vi "Get SysDef Path.vi"(11 "Scalar Channels Testing in":refnum<class "FPGA Addon Test Class.lvclass">) -> (2 "SysDef Path":path, 3 "Scalar Channels Testing out":refnum<class "FPGA Addon Test Class.lvclass">)   [LabVIEW 2019, in "FPGA Addon Test Class.lvclass"]
uses:
  FPGA Addon Test Class.lvclass
  FPGA Addon Test Class.lvclass/FPGA Addon Test Class.ctl
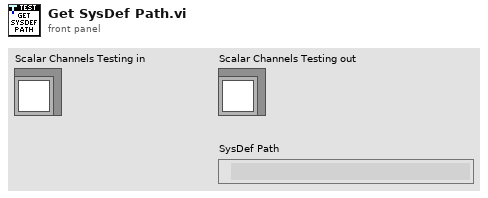
[diagram p1: front panel]
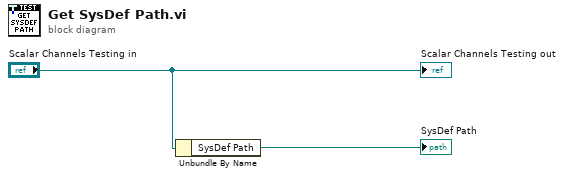
[diagram p0: block diagram]
diagram:
  n1 = Unbundle By Name("Scalar Channels Testing in") -> ("SysDef Path"=→"SysDef Path":path)
  "Scalar Channels Testing out" <- "Scalar Channels Testing in"
